vi "sourcemeter and multimeter2.vi"() -> ()   [LabVIEW 2018]
panel:
  out "output array":dbl[](array[numeric])
  in  "input voltage":dbl[](array[numeric])
  in  "String 2":string="v_dn_21July.lvm"
  in  "String1":string="N_2205_pressure_"
  in  "File Save Folder":path=path "D:/Soumen/OrbitalShaker/Pressure measurement/2205 particles/Run_21July/heating"
  in  "File save - yes/ no?":bool
  in  "For loop count":i32=1000
  in  "format string":string="%0.2f"
  out "Save File Path":path
  out "Reading Result":string
  out "error out":T1
  out "value":dbl
  out "Waveform Chart":dbl(graph)
  in  "error in":T1
  in  "stop":bool
  out "Measure loop":i32
  in  "function (Vdc:1)":u16(ring)=1 items=["ac voltage", "dc voltage", "2-wire resistance", "4-wire resistance", "ac current", "dc current", "frequency", "temperature"]
  in  "GPIB Address":string="16"
  out "Voltage Loop":i32
  out "Set Voltage":string
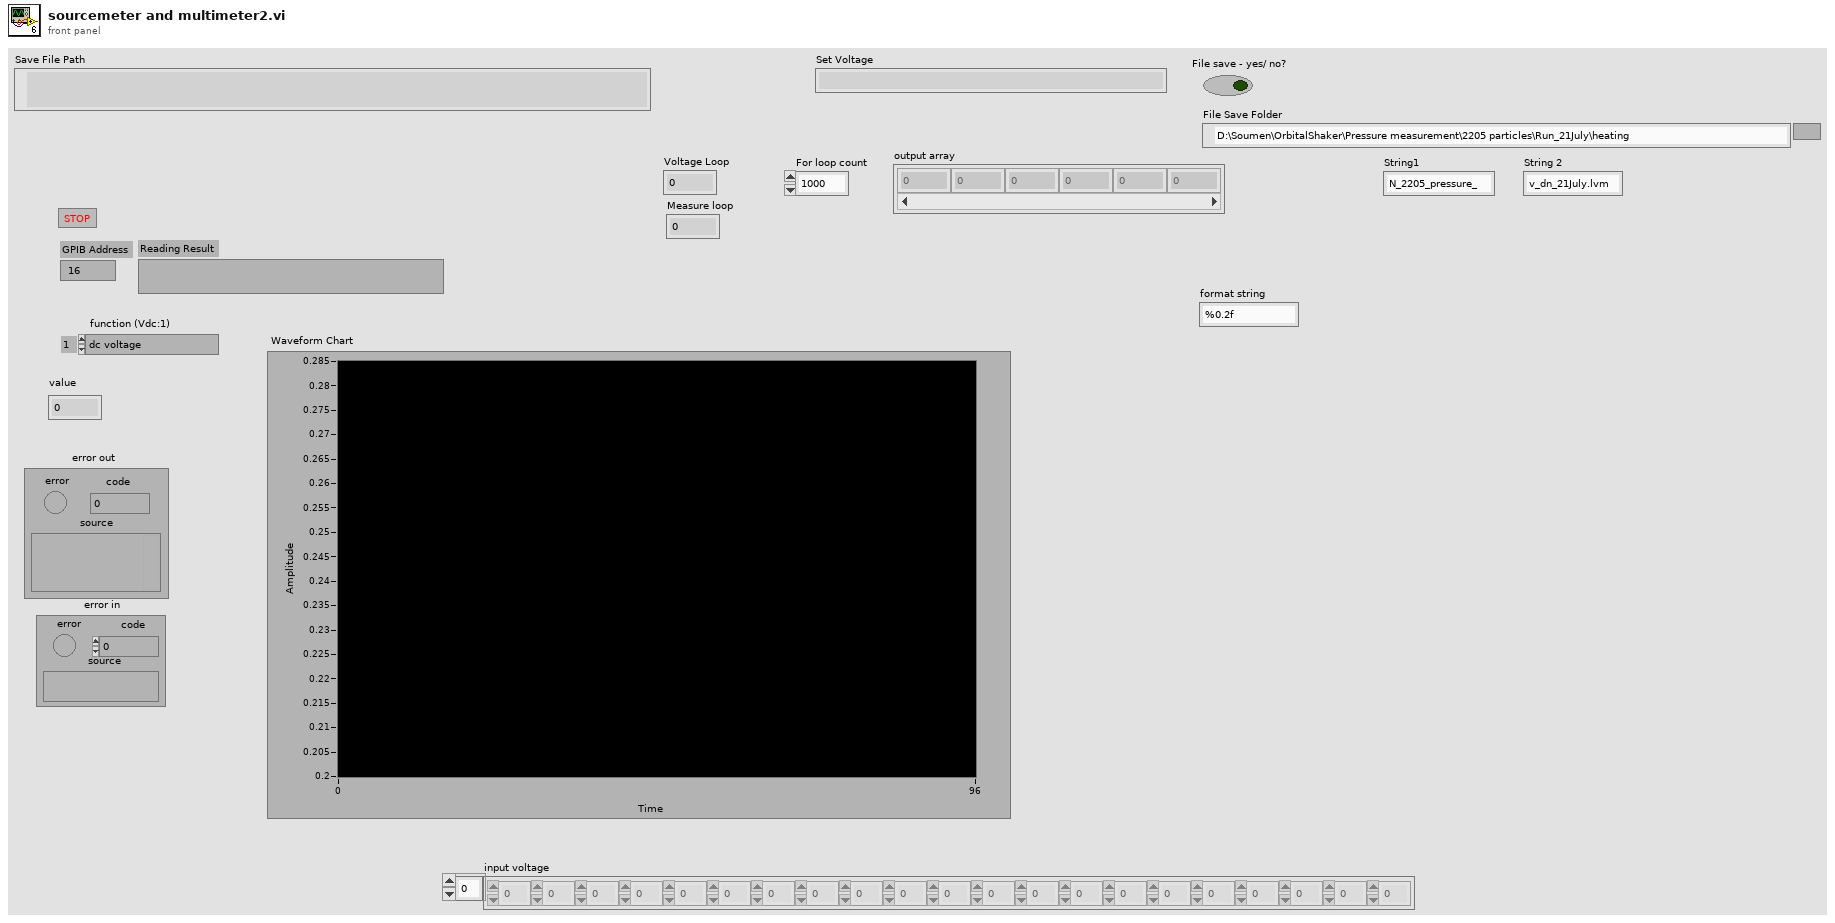
[diagram p1: front panel]
types:
  T1 = cluster{"error":bool, "code":i32, "source":string}
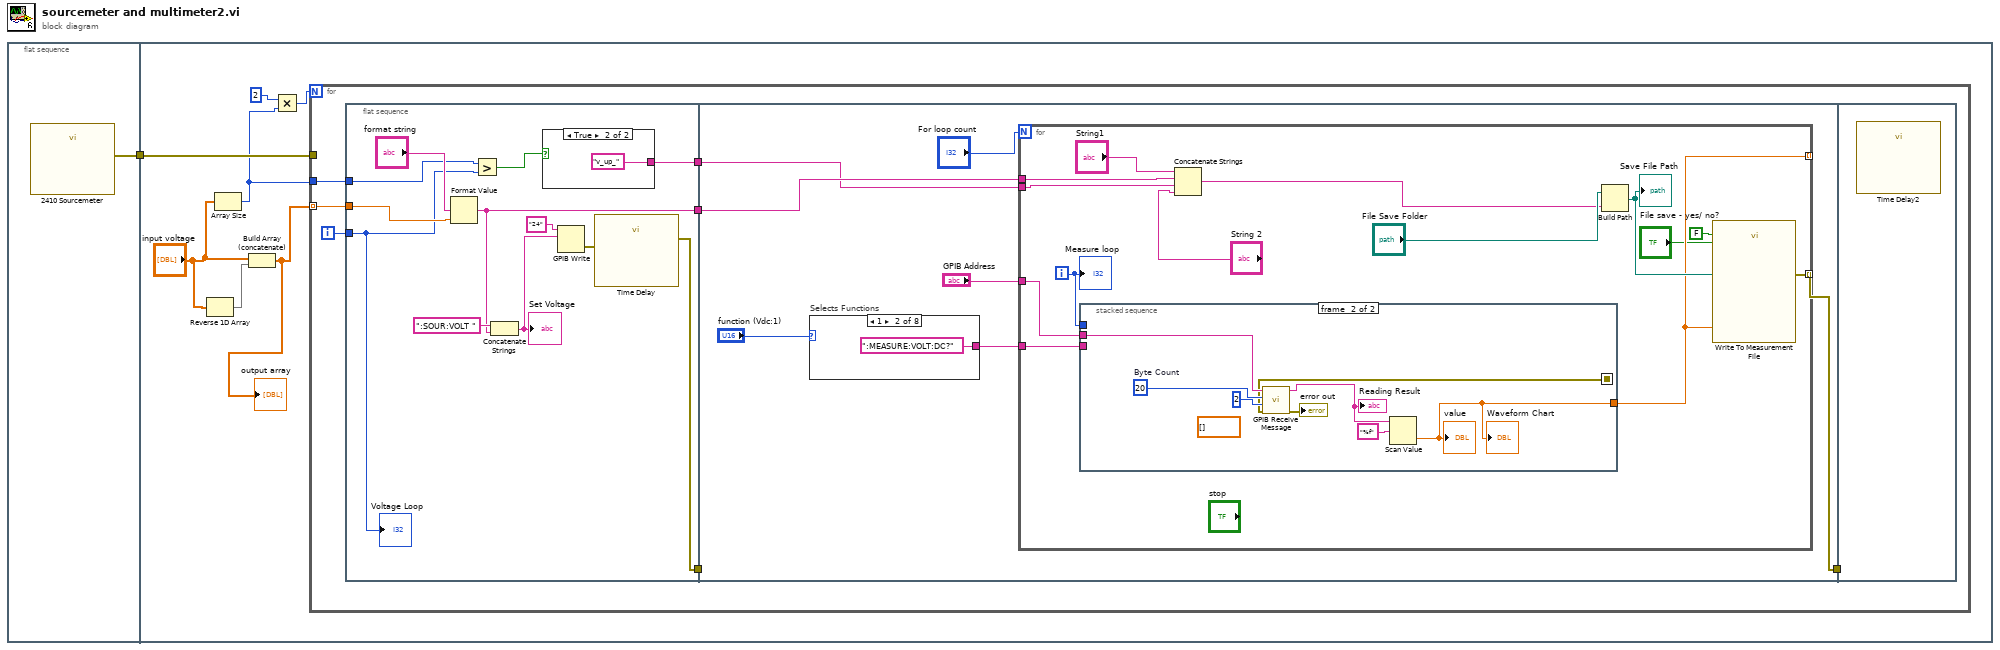
[diagram p0: block diagram]
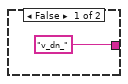
[diagram p2: hidden frame]
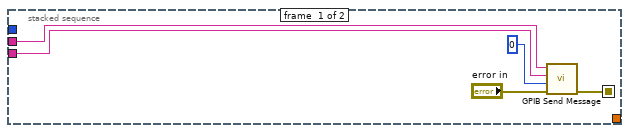
[diagram p3: hidden frame]
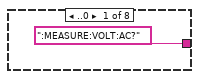
[diagram p4: hidden frame]
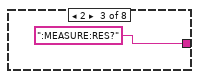
[diagram p5: hidden frame]
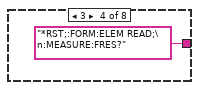
[diagram p6: hidden frame]
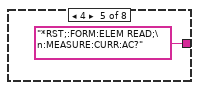
[diagram p7: hidden frame]
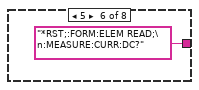
[diagram p8: hidden frame]
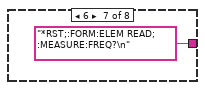
[diagram p9: hidden frame]
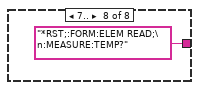
[diagram p10: hidden frame]
diagram:
  n1 = flat-sequence {
    tunnel: [w2] -> w1
    tunnel: w1 -> [w9]
    frame #0 {
      n2 = call "2410 Sourcemeter"() -> ("error out"=w2:errorcluster)  [unwired: 26 in, 1 out]
    }
    frame #1 {
      n3 = Reverse 1D Array(array="input voltage") -> (reversed array=w6:dbl[])
      n4 = Array Size(array="input voltage") -> (size(s)=w3:i32)
      n5 = Build Array (concatenate)("input voltage", w6) -> (w5:dbl[])
      "output array" <- w5
      n6 = Multiply(x=2, y=w3) -> (x*y=w8:i32)
      n7 = for {
        N: w8 -> [_]
        tunnel: w9 -> [_]
        tunnel: w5 -> [w12] mode=indexing
        tunnel: w3 -> [w11]
        i -> [w16]
        n8 = flat-sequence {
          tunnel: w16 -> [w19]
          tunnel: [w24] -> w15
          tunnel: [w22] -> w13
          tunnel: w12 -> [w21]
          tunnel: w11 -> [w20]
          tunnel: [w17] -> w10
          tunnel: w15 -> [_]
          tunnel: [w33] -> w14
          tunnel: w13 -> [w32]
          tunnel: w10 -> [w31]
          tunnel: w14 -> [_]
          frame #0 {
            n9 = Format Value(format string="format string", value (0)=w21) -> (output string=w22:string)  [unwired: 1 in]
            n10 = Greater?(x=w20, y=w19) -> (0:w18:bool)
            n11 = Concatenate Strings(":SOUR:VOLT ", w22) -> (w23:string)
            "Set Voltage" <- w23
            n12 = case shown="True" w18 {
              tunnel: ["v_dn_" "v_up_"] -> w17
              frame False {
              }
              frame True {
              }
            }
            n13 = GPIB Write(0:"24" ("address string"), 1:w23) -> (6:w25:errorcluster)  [unwired: 3 in, 1 out]
            n14 = call "Time Delay"("error in (no error)"=w25) -> ("error out"=w24:errorcluster)  [unwired: 10 in]
            "Voltage Loop" <- w19
          }
          frame #1 {
            n15 = case "Selects Functions" shown="1" "function (Vdc:1)" {
              tunnel: [":MEASURE:VOLT:AC?" ":MEASURE:VOLT:DC?" ":MEASURE:RES?" "*RST;:FORM:ELEM READ;\n:MEASURE:FRES?" "*RST;:FORM:ELEM READ;\n:MEASURE:CURR:AC?" "*RST;:FORM:ELEM READ;\n:MEASURE:CURR:DC?" "*RST;:FORM:ELEM READ; :MEASURE:FREQ?\n" "*RST;:FORM:ELEM READ;\n:MEASURE:TEMP?"] -> w35
              frame ..0 {
              }
              frame 1 {
              }
              frame 2 {
              }
              frame 3 {
              }
              frame 4 {
              }
              frame 5 {
              }
              frame 6 {
              }
              frame 7.. {
              }
            }
            n16 = for {
              N: "For loop count" -> [_]
              tunnel: "GPIB Address" -> [w51]
              tunnel: w35 -> [w50]
              tunnel: [w42] -> _ mode=indexing
              tunnel: [w48] -> w33 mode=indexing
              tunnel: w32 -> [w40]
              tunnel: w31 -> [w39]
              i -> [w49]
              n17 = stacked-sequence {
                seq-local: [w52 _] -> [_ w61]
                tunnel: w51 -> [w56 w64]
                tunnel: w50 -> [w53 _]
                tunnel: w49 -> [_ _]
                tunnel: [_ w57] -> w42
                frame #0 {
                  n18 = call "GPIB Send Message.vi"("address string"=w56, "write buffer"=w53, "write mode (set END:0)"=0, "error in"="error in") -> ("error out"=w52:T1)  [unwired: 3 in, 2 out]
                }
                frame #1 {
                  (unwired) dbl[] [] ("Waveform Graph")
                  w63 = 20  # Byte Count
                  n19 = call "GPIB Receive Message.vi"("address string"=w64, "byte count"=w63, "read mode"=2, "error in"=w61) -> ("read buffer"=w59:string, "error out"=→"error out":T1)  [unwired: 3 in, 1 out]
                  "Reading Result" <- w59
                  n20 = Scan Value(string=w59, format string="%f") -> (value=w57:dbl)  [unwired: 1 in, 1 out]
                  "value" <- w57
                  "Waveform Chart" <- w57
                }
              }
              n21 = Concatenate Strings("String1", w40, w39, "String 2") -> (w45:string)
              n22 = Build Path(base path="File Save Folder", name or relative path=w45) -> (appended path=w44:path)
              "Save File Path" <- w44
              n23 = call "Write To Measurement File"("Signals"=w42, "Reset"=FALSE, "Enable"="File save - yes/ no?", "Filename"=w44) -> ("error out"=w48:errorcluster)  [unwired: 13 in, 2 out]
              "Measure loop" <- w49
            }
          }
          frame #2 {
            n24 = call "Time Delay2"() -> ()  [unwired: 11 in, 1 out]
          }
        }
      }
    }
  }
